vi "setRunState.vi"(8 "error in (no error)":errorcluster, 10 "Runstate":bool, 11 "FgenNiPxi in":refnum<class "ArbNi.lvclass">) -> (0 "error out":errorcluster, 3 "FgenNiPxi out":refnum<class "ArbNi.lvclass">)   [LabVIEW 2023, in "ArbNi.lvclass"]
uses:
  ArbNi.lvclass
  ArbNi.lvclass/ArbNi.ctl
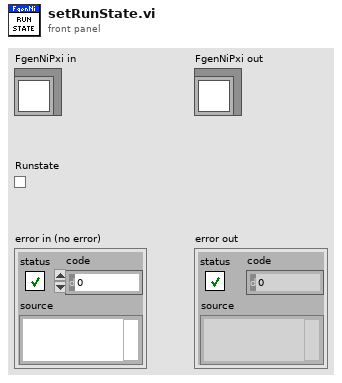
[diagram p1: front panel]
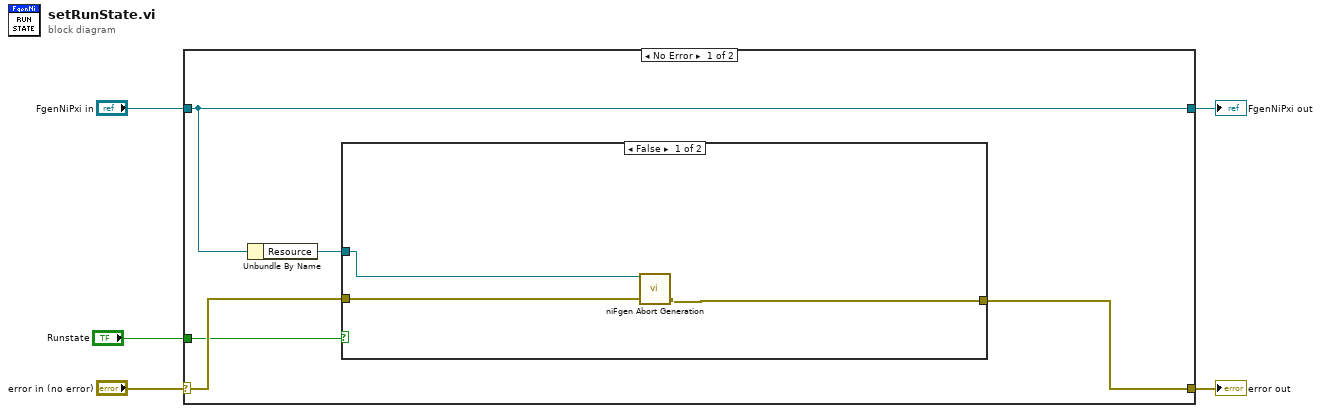
[diagram p0: block diagram]
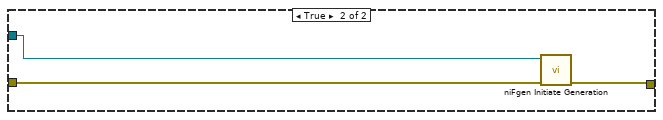
[diagram p2: hidden frame]
diagram:
  n1 = case shown="No Error" "error in (no error)" {
    selector: "error in (no error)" -> [w8 w18]
    tunnel: [w7 w18] -> w4
    tunnel: [w10 w17] -> w2
    tunnel: "FgenNiPxi in" -> [w10 w17]
    tunnel: "Runstate" -> [w6 _]
    frame No Error {
      n2 = Unbundle By Name(w10) -> ("Resource"=w9:refnum<k15>)
      n3 = case shown="False" w6 {
        tunnel: w8 -> [w13 w14]
        tunnel: w9 -> [w11 w16]
        tunnel: [w12 w15] -> w7
        frame False {
          n4 = call <instrlib>:"niFgen Abort Generation.vi"("error in (no error)"=w13, "Instrument Handle"=w11) -> ("error out"=w12:errorcluster)  [unwired: 8 in, 1 out]
        }
        frame True {
          n5 = call <instrlib>:"niFgen Initiate Generation.vi"("error in (no error)"=w14, "Instrument Handle"=w16) -> ("error out"=w15:errorcluster)  [unwired: 8 in, 1 out]
        }
      }
    }
    frame Error {
    }
  }
  "error out" <- w4
  "FgenNiPxi out" <- w2
